vi "Create.vi"(7 "options":T13, 8 "error in (no error)":errorcluster, 11 "Device Item Ref":T18=18446744073709551615 format="%.0x") -> (0 "error out":errorcluster, 2 "framework configuration":T1, 3 "VeriStand Framework":refnum<class "VeriStand Data Sharing Framework.lvclass">)   [LabVIEW 2017, in "Data Sharing Framework Engine.lvlib" / "VeriStand Data Sharing Framework.lvclass"]
uses:
  VeriStand Data Sharing Framework.lvclass
  <vilib>/NI Veristand/Custom Device API/Custom Device Item Ref.ctl
  DSF Core.lvlibp/Engine/Classes/Framework/Framework Options.ctl
  DSF Core.lvlibp/Engine/Typedefs/FIFO Flags.ctl
  DSF Core.lvlibp/Engine/Classes/Thread/Thread Options.ctl
  DSF Core.lvlibp/Engine/Typedefs/Plugin Flags.ctl
  DSF Core.lvlibp/Engine/Typedefs/Performance Options.ctl
  DSF Core.lvlibp/DSF Configuration API/Public/Controls/DSF Engine Framework Configuration.ctl
  DSF Core.lvlibp/DSF Configuration API/Public/Controls/DSF Engine Plugin Configuration.ctl
  DSF Core.lvlibp/DSF Configuration API/Public/Controls/DSF Timing Info.ctl
  DSF Core.lvlibp/DSF Configuration API/Public/Controls/DSF Engine Plugin Thread Configuration.ctl
  DSF Core.lvlibp/DSF Configuration API/Public/Controls/DSF Settings Info.ctl
  DSF Core.lvlibp/DSF Configuration API/Public/Controls/DSF Engine Transfer Group Configuration.ctl
  DSF Core.lvlibp/DSF Configuration API/Public/Controls/DSF Direction.ctl
  DSF Core.lvlibp/DSF Configuration API/Public/Controls/DSF Engine Transfer Configuration.ctl
  DSF Core.lvlibp/DSF Configuration API/Public/Controls/DSF Byte Order.ctl
  DSF Core.lvlibp/DSF Configuration API/Public/Controls/DSF Engine Channel Configuration.ctl
  DSF Core.lvlibp/DSF Configuration API/Public/Controls/DSF Data Type.ctl
  DSF Core.lvlibp/DSF Configuration API/Public/Controls/DSF Timeout Behavior.ctl
  VeriStand Data Sharing Framework.lvclass/VeriStand Data Sharing Framework.ctl
  <vilib>/NI Veristand/Custom Device API/Get Item Property (Dependent File).vi
  <vilib>/NI Veristand/Custom Device API/Custom Device API.lvlib
  DSF Core.lvlibp/DSF Configuration API/Configuration Session.lvclass
  DSF Core.lvlibp
  DSF Core.lvlibp/Engine/Classes/Framework/Framework.lvclass
  DSF Core.lvlibp/Engine/Classes/Status/Performance.lvclass
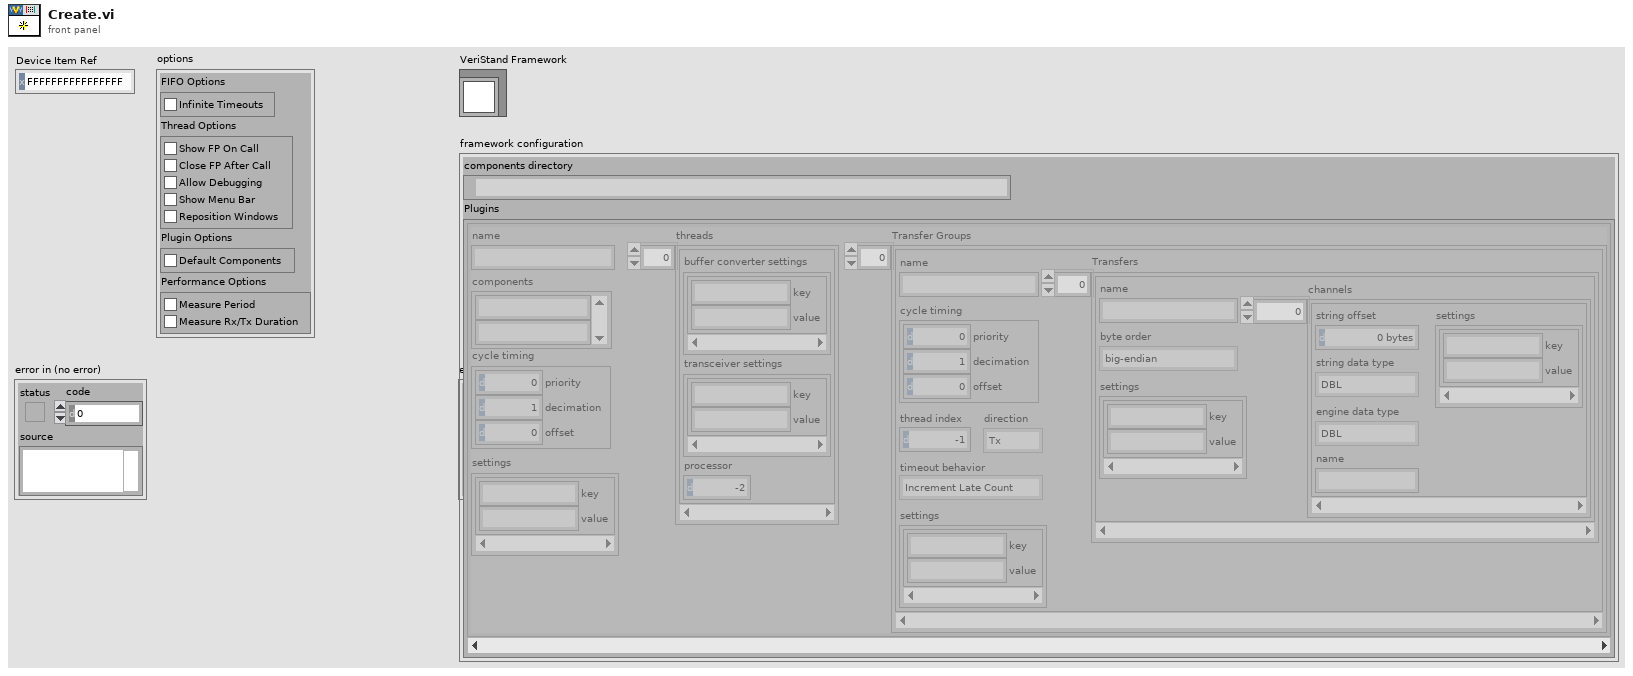
[diagram p1: front panel]
types:
  T1 = typedef "DSF Core.lvlibp/DSF Engine Framework Configuration.ctl" = cluster{"components directory":path, "Plugins":T2[]}
  T2 = typedef "DSF Core.lvlibp/DSF Engine Plugin Configuration.ctl" = cluster{"name":string, "components":string[], "cycle timing":T3, "threads":T4[], "Transfer Groups":T6[], "settings":T5}
  T3 = typedef "DSF Core.lvlibp/DSF Timing Info.ctl" = cluster{"priority":u64, "decimation":u64, "offset":u64}
  T4 = typedef "DSF Core.lvlibp/DSF Engine Plugin Thread Configuration.ctl" = cluster{"buffer converter settings":T5, "transceiver settings":T5, "processor":i32}
  T5 = typedef "DSF Core.lvlibp/DSF Settings Info.ctl" = cluster{"key":string, "value":string}[]
  T6 = typedef "DSF Core.lvlibp/DSF Engine Transfer Group Configuration.ctl" = cluster{"name":string, "direction":T7, "cycle timing":T3, "thread index":i32, "settings":T5, "Transfers":T8[], "timeout behavior":T12}
  T7 = typedef "DSF Core.lvlibp/DSF Direction.ctl" = enum8{"Tx", "Rx"}
  T8 = typedef "DSF Core.lvlibp/DSF Engine Transfer Configuration.ctl" = cluster{"name":string, "byte order":T9, "settings":T5, "channels":T10[]}
  T9 = typedef "DSF Core.lvlibp/DSF Byte Order.ctl" = enum8{"big-endian", "little-endian"}
  T10 = typedef "DSF Core.lvlibp/DSF Engine Channel Configuration.ctl" = cluster{"string offset":u64, "string data type":T11, "engine data type":T11, "name":string, "settings":T5}
  T11 = typedef "DSF Core.lvlibp/DSF Data Type.ctl" = enum8{"Bool", "SGL", "DBL", "I8", "I16", "I32", "I64", "U8", "U16", "U32", "U64"}
  T12 = typedef "DSF Core.lvlibp/DSF Timeout Behavior.ctl" = enum16{"Increment Late Count", "Throw Error"}
  T13 = typedef "DSF Core.lvlibp/Framework.lvclass/Framework Options.ctl" = cluster{"FIFO Options":T14, "Thread Options":T15, "Plugin Options":T16, "Performance Options":T17}
  T14 = typedef "DSF Core.lvlibp/FIFO Flags.ctl" = cluster{"Infinite Timeouts":bool}
  T15 = typedef "DSF Core.lvlibp/Thread Options.ctl" = cluster{"Show FP On Call":bool, "Close FP After Call":bool, "Allow Debugging":bool, "Show Menu Bar":bool, "Reposition Windows":bool}
  T16 = typedef "DSF Core.lvlibp/Plugin Flags.ctl" = cluster{"Default Components":bool}
  T17 = typedef "DSF Core.lvlibp/Performance.lvclass/Performance Options.ctl" = cluster{"Measure Period":bool, "Measure Rx/Tx Duration":bool}
  T18 = typedef "Custom Device API.lvlib/Custom Device Item Ref.ctl" = u64
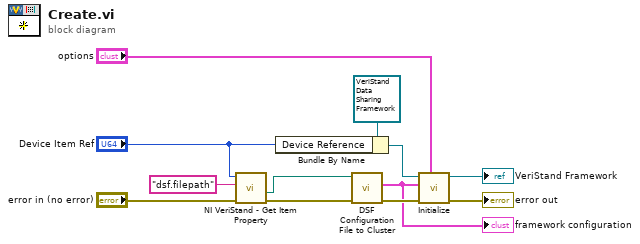
[diagram p0: block diagram]
diagram:
  n1 = call-poly <vilib>:"NI VeriStand - Get Item Property.vi"("error in (no error)"="error in (no error)", "Property Name"="dsf.filepath", "Item Ref in"="Device Item Ref") -> ("error out"=w2:errorcluster, "Path"=w3:path)  [unwired: 4 in, 3 out]
  n2 = Bundle By Name(cluster=refnum<class "VeriStand Data Sharing Framework.lvclass"> refnum ("VeriStand Data Sharing Framework out"), "Device Reference"="Device Item Ref") -> (w8:refnum<class "VeriStand Data Sharing Framework.lvclass">)
  n3 = call "DSF Configuration File to Cluster.vi"("error in (no error)"=w2, "dsf configuration file path"=w3) -> ("error out"=w9:errorcluster, "framework configuration out"=w7:T1)  [unwired: 7 in, 1 out]
  "framework configuration" <- w7
  n4 = call-dynamic "Initialize.vi"("options"="options", "error in (no error)"=w9, "framework configuration"=w7, "VeriStand Data Sharing Framework in"=w8) -> ("error out"=→"error out":errorcluster, "VeriStand Data Sharing Framework out"=→"VeriStand Framework":refnum<class "VeriStand Data Sharing Framework.lvclass">)  [unwired: 6 in]
